vi "Intensityduplex.vi"(0 "Enum":T1(ring), 1 "Image In":T2, 2 "add string":string, 3 "error in":errorcluster, 4 "title":string) -> (5 "Image Duplicate (out)":T2, 6 "title out":string)   [LabVIEW 2009]
uses:
  <vilib>/vision/Image Controls.llb/IMAQ Image.ctl
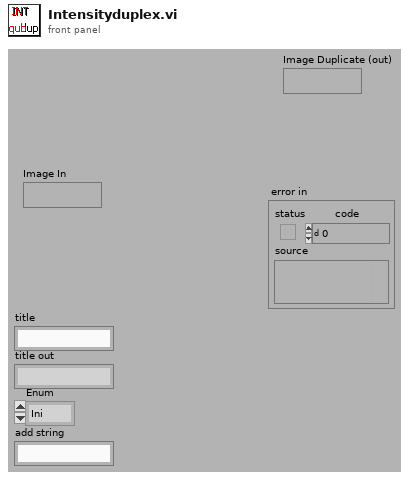
[diagram p1: front panel]
types:
  T1 = enum16{"Ini", "Get", "Set", "Refresh", "dump", "move", "name"}
  T2 = typedef "IMAQ Image.ctl" = refnum<image>
  T3 = enum16{"Ini", "Get", "Set", "Refresh", "dump", "move"}
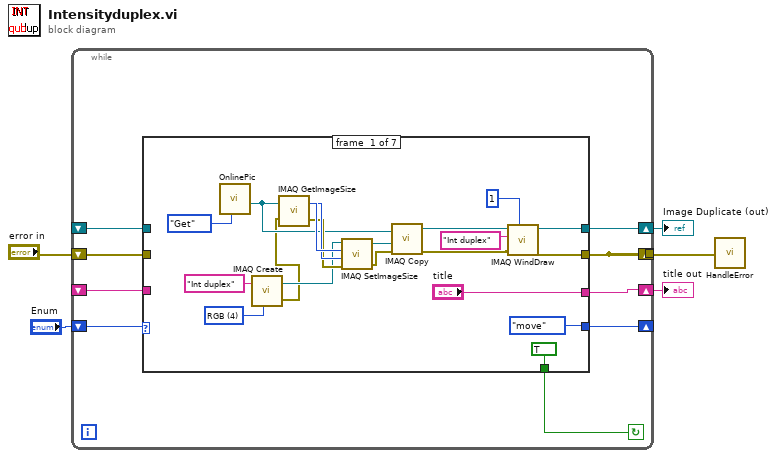
[diagram p0: block diagram]
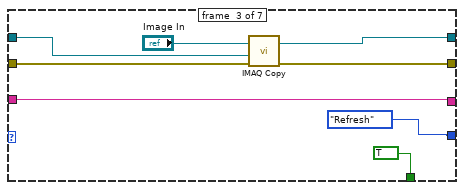
[diagram p3: hidden frame]
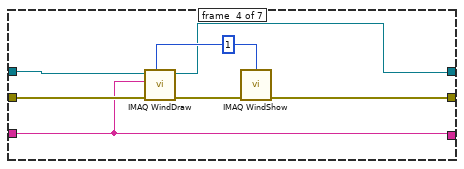
[diagram p4: hidden frame]
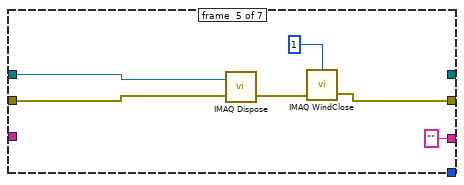
[diagram p5: hidden frame]
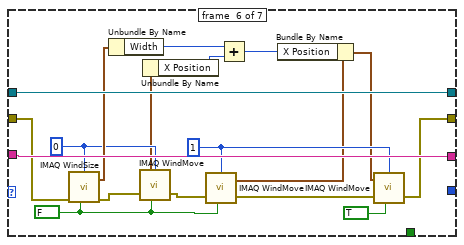
[diagram p6: hidden frame]
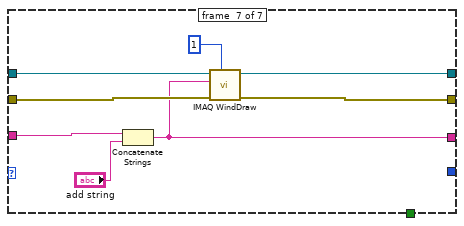
[diagram p7: hidden frame]
diagram:
  n1 = while {
    shift-right: [w14] -> w5
    shift-left: _ -> [w13]
    shift-right: [w8] -> _
    shift-left: "Enum" -> [w11]
    shift-right: [w9] -> w1
    shift-left: "error in" -> [w10]
    tunnel: [w9] -> _
    shift-right: [w6] -> w3
    shift-left: _ -> [w7]
    stop <- w12 continue-if-true
    n2 = case shown="\"Ini\"" w11 {
      tunnel: [w27 w36 w40 w46 _ w74 w81] -> w14
      tunnel: [w26 _ w41 w50 w52 w62 w80] -> w9
      tunnel: w13 -> [_ w36 w38 w47 w55 w74 w82]
      tunnel: [TRUE _ TRUE _ _ _ _] -> w12
      tunnel: w10 -> [_ _ w42 w49 w56 w73 w83]
      tunnel: [T3."move" ("Enum") _ enum16{"Ini", "Get", "Set", "Refresh"}."Refresh" ("Enum") _ _ _ _] -> w8
      tunnel: w7 -> [_ w35 w39 w45 _ w75 w76]
      tunnel: ["title" w35 w39 w45 "" ("title") w75 w78] -> w6
      frame #0 {
        w29 = u32 4 items=["8 bits", "16 bits", "Float", "Complex", "RGB", "HSL"] ("Image Type")
        n3 = call "OnlinePic.vi"("action"=enum16{"Get", "Set", "Change", "ini"}."Get" ("Enum")) -> ("Image Out (duplicate)"=w19:T2)  [unwired: 6 in, 4 out]
        n4 = call "IMAQ Create"("Image Name"="Int duplex", "Image Type"=w29) -> ("New Image"=w18:T2, "error out"=w16:errorcluster)  [unwired: 3 in]
        n5 = call "IMAQ GetImageSize"("Image"=w19, "error in (no error)"=w16) -> ("Y Resolution"=w21:i32, "X Resolution"=w22:i32, "error out"=w20:errorcluster)  [unwired: 2 in]
        n6 = call "IMAQ SetImageSize"("error in (no error)"=w20, "Y Resolution"=w21, "X Resolution"=w22, "Image"=w18) -> ("error out"=w15:errorcluster, "Image Out"=w17:T2)  [unwired: 1 in]
        n7 = call "IMAQ Copy"("error in (no error)"=w15, "Image Dst"=w17, "Image Src"=w19) -> ("error out"=w33:errorcluster, "Image Dst Out"=w31:T2)  [unwired: 3 in]
        n8 = call "IMAQ WindDraw"("Window Number (0...15)"=1, "error in (no error)"=w33, "Title"="Int duplex", "Image"=w31) -> ("error out"=w26:errorcluster, "Image Out (duplicate)"=w27:T2)  [unwired: 6 in]
      }
      frame #1 {
      }
      frame #2 {
        n9 = call "IMAQ Copy"("error in (no error)"=w42, "Image Dst"=w38, "Image Src"="Image In") -> ("error out"=w41:errorcluster, "Image Dst Out"=w40:T2)  [unwired: 3 in]
      }
      frame #3 {
        w51 = 1 ("Window Number (0...15)")
        n10 = call "IMAQ WindDraw"("Window Number (0...15)"=w51, "error in (no error)"=w49, "Title"=w45, "Image"=w47) -> ("error out"=w48:errorcluster, "Image Out (duplicate)"=w46:T2)  [unwired: 6 in]
        n11 = call "IMAQ WindShow"("error in (no error)"=w48, "Window Number (0...15)"=w51) -> ("error out"=w50:errorcluster)  [unwired: 4 in, 2 out]
      }
      frame #4 {
        n12 = call "IMAQ Dispose"("Image"=w55, "error in (no error)"=w56) -> ("error out"=w54:errorcluster)  [unwired: 4 in]
        n13 = call "IMAQ WindClose"("Window Number (0...15)"=1, "error in (no error)"=w54) -> ("error out"=w52:errorcluster)  [unwired: 4 in]
      }
      frame #5 {
        w67 = FALSE ("Get/Set Status? (Set)")
        w65 = 1 ("Window Number (0...15)")
        w70 = 0 ("Window Number")
        n14 = call "IMAQ WindSize"("error in (no error)"=w73, "Get/Set Status? (Set)"=w67, "Window Number"=w70) -> ("error out"=w72:errorcluster, "Width & Height out"=w71:cluster{"Width":i32, "Height":i32})  [unwired: 3 in, 1 out]
        n15 = Unbundle By Name(w71) -> ("Width"=w59:i32)
        n16 = call "IMAQ WindMove"("Window Number (0...15)"=w70, "Get/Set Status? (Set)"=w67, "error in (no error)"=w72) -> ("Coordinates (screen)"=w61:cluster{"X Position":i32, "Y Position":i32}, "error out"=w69:errorcluster)  [unwired: 2 in]
        n17 = Unbundle By Name(w61) -> ("X Position"=w60:i32)
        n18 = call "IMAQ WindMove"("Window Number (0...15)"=w65, "Get/Set Status? (Set)"=w67, "error in (no error)"=w69) -> ("Coordinates (screen)"=w64:cluster{"X Position":i32, "Y Position":i32}, "error out"=w68:errorcluster)  [unwired: 2 in]
        n19 = Add(x=w59, y=w60) -> (x+y=w58:i32)
        n20 = Bundle By Name(cluster=w64, "X Position"=w58) -> (w63:cluster{"X Position":i32, "Y Position":i32})
        n21 = call "IMAQ WindMove"("Window Number (0...15)"=w65, "Coordinates (screen)"=w63, "Get/Set Status? (Set)"=TRUE, "error in (no error)"=w68) -> ("error out"=w62:errorcluster)  [unwired: 1 in, 1 out]
      }
      frame #6 {
        n22 = Concatenate Strings(w76, "add string") -> (w78:string)
        n23 = call "IMAQ WindDraw"("Window Number (0...15)"=1, "error in (no error)"=w83, "Title"=w78, "Image"=w82) -> ("error out"=w80:errorcluster, "Image Out (duplicate)"=w81:T2)  [unwired: 6 in]
      }
    }
  }
  "Image Duplicate (out)" <- w5
  "title out" <- w3
  n24 = call "HandleError.vi"("error in (no error)"=w1) -> ()
